vi "Check Waveform Group Channel Name.vi"(8 "error in (no error)":errorcluster, 9 "Group Name":string, 10 "Channel Name":string, 11 "TDMS File In":refnum<k34>) -> (0 "error out":errorcluster, 3 "TDMS File Out":refnum<k34>)   [LabVIEW 2013, in "Agilent 90000 Series.lvlib"]
doc: "Checks whether the TDMS file has the specified group name and channel name."
uses:
  Agilent 90000 Series.lvlib
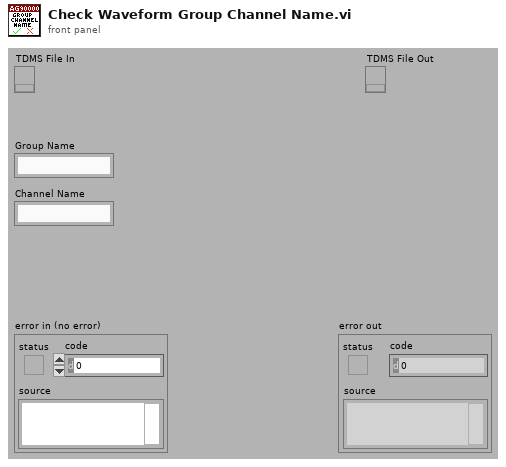
[diagram p1: front panel]
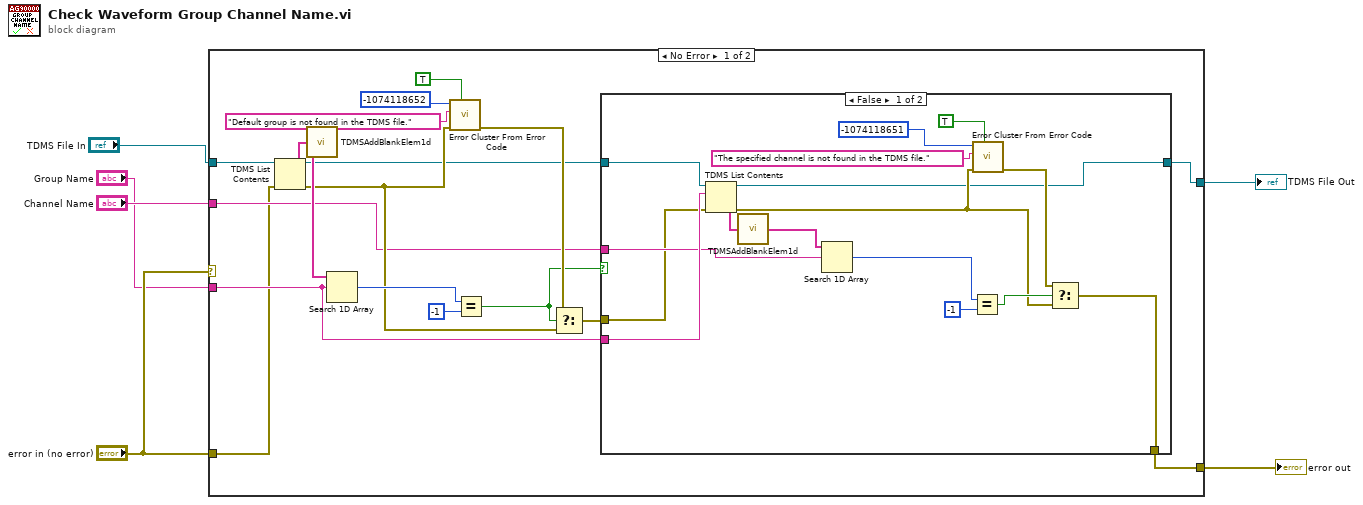
[diagram p0: block diagram]
diagram:
  n1 = case shown="No Error" "error in (no error)" {
    tunnel: "TDMS File In" -> [w23 w43]
    tunnel: "Channel Name" -> [w12 _]
    tunnel: [w24 w44] -> w5
    tunnel: "error in (no error)" -> [w8 w44]
    tunnel: [w9 w43] -> w4
    tunnel: "Group Name" -> [w11 _]
    frame No Error {
      n2 = TDMS List Contents(4:w8, 7:w23) -> (0:w15:errorcluster, 2:w7:string[], 3:w13:refnum<k34>)  [unwired: 1 in, 1 out]
      n3 = call <vilib>:"TDMSAddBlankElem1d.vi"("input string array"=w7) -> ("output string array with blank element at the beginning"=w22:string[])
      n4 = Search 1D Array(1D array=w22, element=w11) -> (index of element=w18:i32)  [unwired: 1 in]
      n5 = call <vilib>:"Error Cluster From Error Code.vi"("show call chain? (False)"=TRUE, "error in (no error)"=w15, "error message (\"\")"="Default group is not found in the TDMS file." ("error message (\"\")"), "error code (0)"=-1074118652) -> ("error out"=w16:errorcluster)  [unwired: 5 in]
      n6 = Equal?(x=w18, y=-1) -> (x = y?=w14:bool)
      n7 = Select(t=w16, s=w14, f=w15) -> (s? t:f=w10:errorcluster)
      n8 = case shown="False" w14 {
        tunnel: [w27 w42] -> w24
        tunnel: w12 -> [w37 _]
        tunnel: w13 -> [w40 w41]
        tunnel: w11 -> [w39 _]
        tunnel: w10 -> [w34 w42]
        tunnel: [w26 w41] -> w9
        frame False {
          n9 = TDMS List Contents(4:w34, 6:w39, 7:w40) -> (0:w28:errorcluster, 1:w25:string[], 3:w26:refnum<k34>)  [unwired: 1 out]
          n10 = call <vilib>:"TDMSAddBlankElem1d.vi"("input string array"=w25) -> ("output string array with blank element at the beginning"=w38:string[])
          n11 = Search 1D Array(1D array=w38, element=w37) -> (index of element=w35:i32)  [unwired: 1 in]
          n12 = Equal?(x=w35, y=-1) -> (x = y?=w33:bool)
          n13 = call <vilib>:"Error Cluster From Error Code.vi"("show call chain? (False)"=TRUE, "error in (no error)"=w28, "error message (\"\")"="The specified channel is not found in the TDMS file." ("error message (\"\")"), "error code (0)"=-1074118651) -> ("error out"=w29:errorcluster)  [unwired: 5 in]
          n14 = Select(t=w29, s=w33, f=w28) -> (s? t:f=w27:errorcluster)
        }
        frame True {
        }
      }
    }
    frame Error {
    }
  }
  "error out" <- w5
  "TDMS File Out" <- w4
